vi "Mass_2_1_old.vi"() -> ()   [LabVIEW 2020]
uses:
  Support/Controls/Cmd_Mouse Popup.ctl
  Support/Controls/Clst_Initialize Input.ctl
  Support/Controls/Clst_Result inspec.ctl
  Support/Controls/Cmd_Var Data IO.ctl
  Variables/Global_Cal Info.vi
  <vilib>/express/express arith-compare/Formula/XNode/ExpressFormulaBlockNode.xnode
panel:
  in  "일괄\n변경":bool=TRUE
  in  "분동등급":string(combo)
  out "적용?":bool
  in  "다음 버튼":bool
  in  "이전 버튼":bool
  in  "제거":bool
  in  "적용":bool
  out "추가명목값":string caption="명목값"
  in  "추가":bool
  in  "추가문자열":string
  in  "시험분동 추가":i32(listbox)=24
  out "분해능":string caption="저울분해능 (g)"
  out "Data Out":string[][](table)
  out "단위":string
  out "명목질량":string
  in  "기기번호":string
  out "명목값":string
  in  "편심오차":string[][](table) caption="4. 저울 편심오차 시험"
  in  "측정횟수":i32(ring)=5 items=["5회"=5, "10회"=10]
  in  "시험분동밀도":string="8000" caption="분동밀도 (kg/㎤)"
  out "감도분동":string
  out "X=S-T":string[][](table)
  out "공기밀도":string
  out "Header2":string[][](table)
  in  "Measured":string[][](table) caption="3. 저울 지시값"
  out "Weight info":string[][](table) caption="2. 분동식별표기"
  out "Spec":string[][](table)
  in  "시험분동":i32(listbox)=-1
  in  "Spec 변경":bool
  out "제목":string
  out "에러 출력":errorcluster
  out "Condition":string[][](table)
  out "Atm Env":string[][](table) caption="1. 측정환경"
  out "Load?":bool
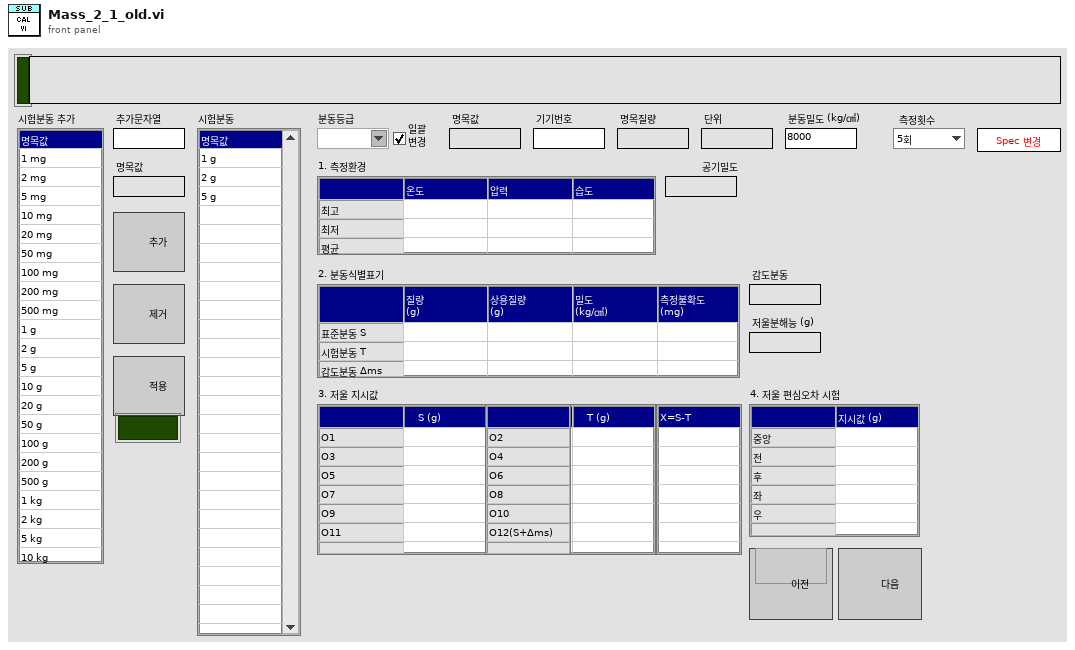
[diagram p1: front panel]
types:
  T1 = typedef "Cmd_Mouse Popup.ctl" = enum16{"활성화", "메뉴선택"}
  T2 = cluster{"Shift":bool, "Ctrl":bool, "Alt":bool, "Cmd":bool, "Opt":bool}
  T3 = typedef "Clst_Initialize Input.ctl" = cluster{"Initialize 1":cluster{"Condition":refnum<vi>[], "Spec":refnum<vi>[], "Measured":refnum<vi>[], "Resolution":refnum<vi>[], "Func_ext":string, "제목":refnum<vi>, "Measured_ADJ":refnum<vi>[]}, "Initialize 2":cluster{"문자열":refnum<vi>[], "콤보박스":refnum<vi>[], "링":refnum<vi>[], "열거형":refnum<vi>[], "테이블":refnum<vi>[], "여러열":refnum<vi>[], "디지털(DBL)":refnum<vi>[], "3D string":refnum<vi>[], "ctrl":refnum<vi>[], "boolean":refnum<vi>[]}}
  T4 = typedef "Cmd_Var Data IO.ctl" = enum16{"Condition", "Condition Default", "Condition_Temp", "Resolution", "Resolution Default", "Resolution Old", "Spec", "Spec Default", "Spec Old", "Spec Temp", "Result", "Result2", "Result3", "Result_Temp", "Result_ADJ", "Result_ADJ2", "STD1", "STD2", "STD3", "STD4", "STD5", "STD Temp", "CMC", "CMC Default"}
  T5 = typedef "Clst_Result inspec.ctl" = cluster{"분해능":string, "문자열 1":string, "문자열 2":string, "숫자형 1":i32, "숫자형 2":i32, "숫자형 3":dbl, "문자배열 1D":string[], "문자배열 2D":string[][], "문자배열 3D":string[][][], "문자배열 4D":string[][][][], "불리언 1D":bool[]}
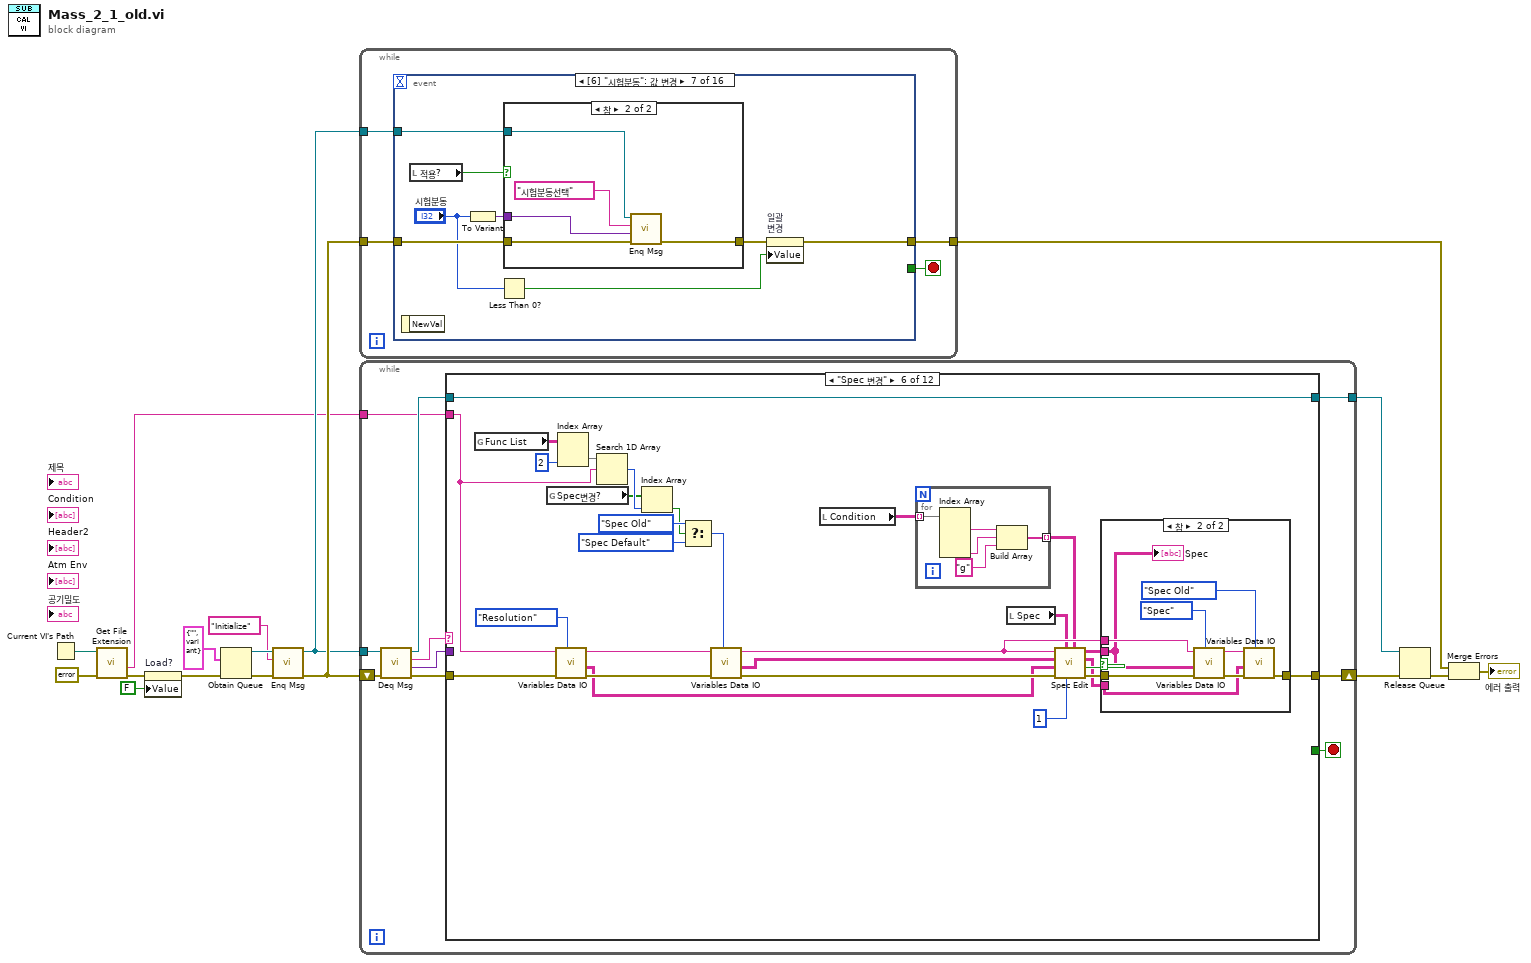
[diagram p0: block diagram]
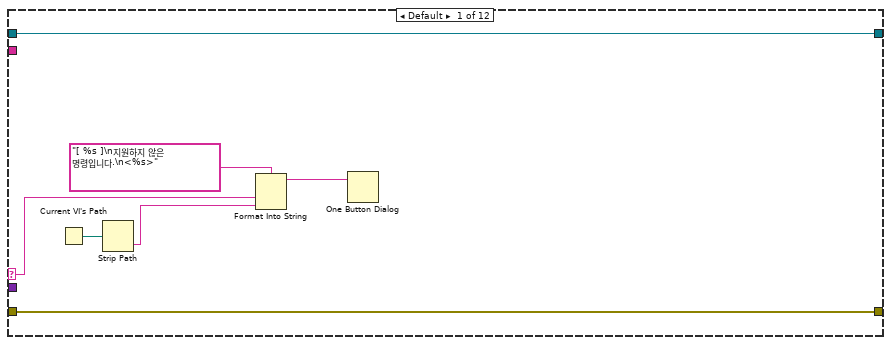
[diagram p2: hidden frame]
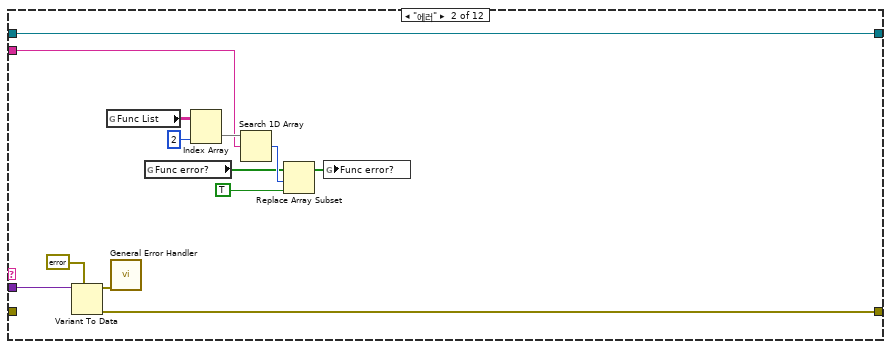
[diagram p3: hidden frame]
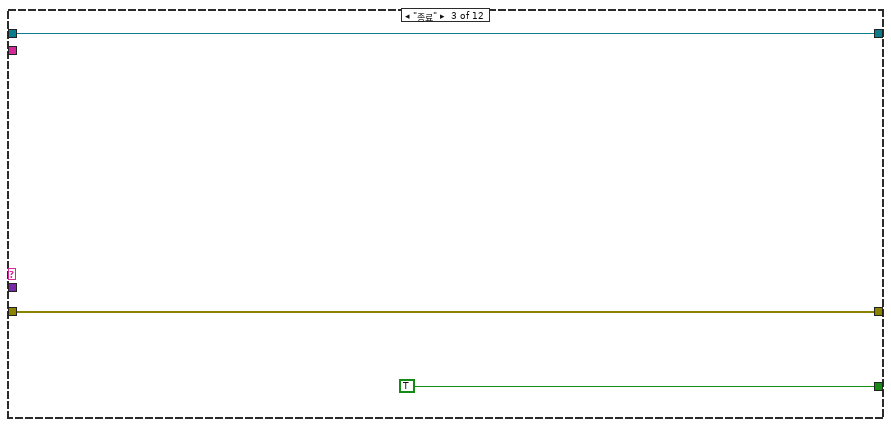
[diagram p4: hidden frame]
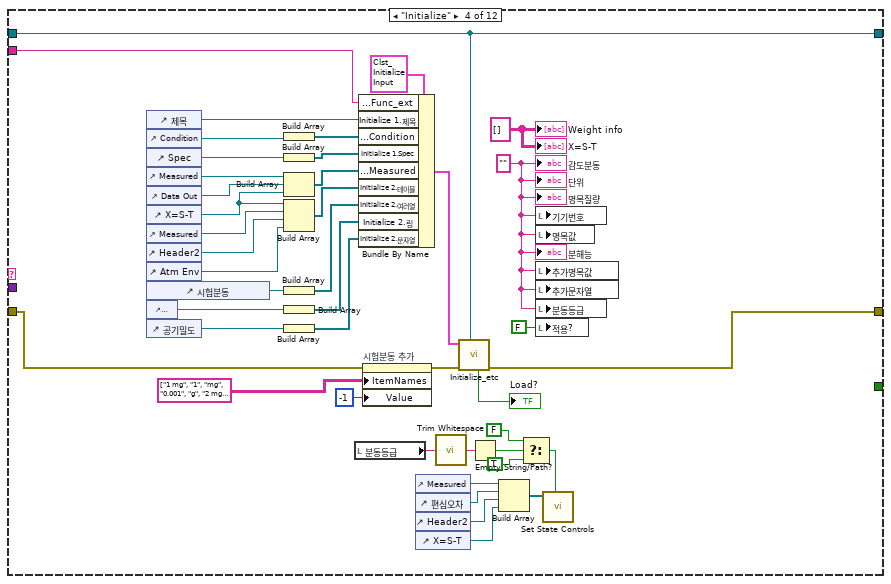
[diagram p5: hidden frame]
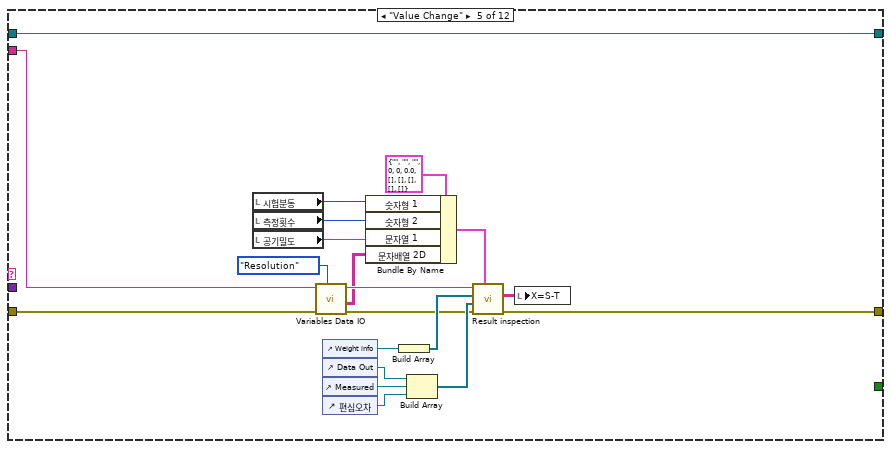
[diagram p6: hidden frame]
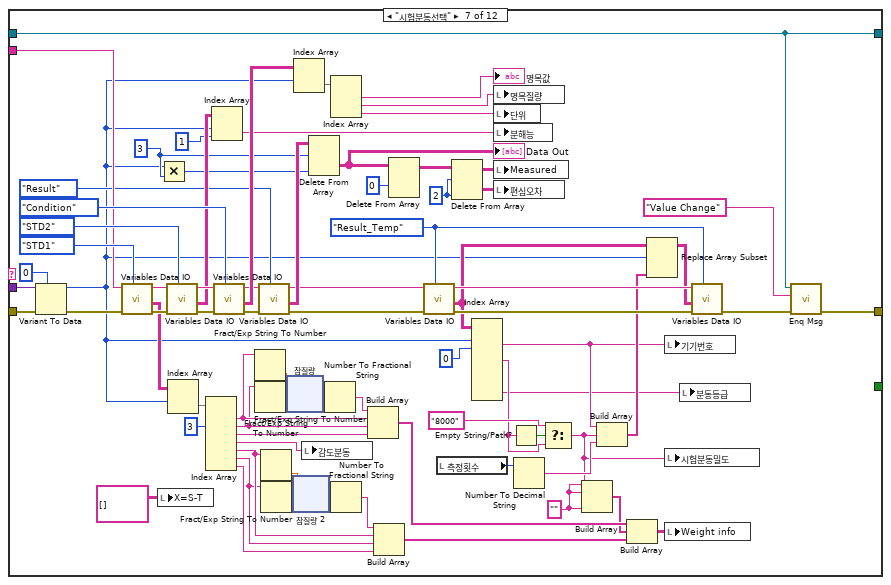
[diagram p8: hidden frame]
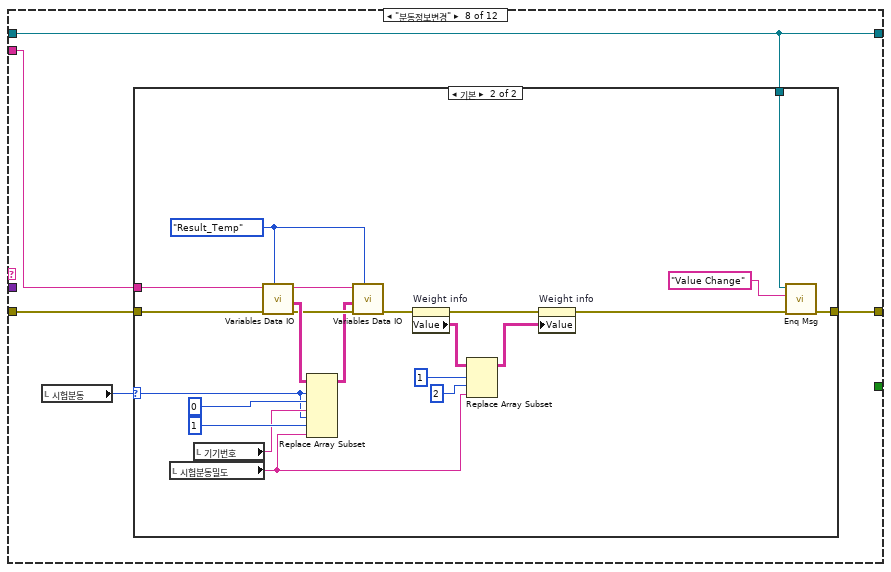
[diagram p9: hidden frame]
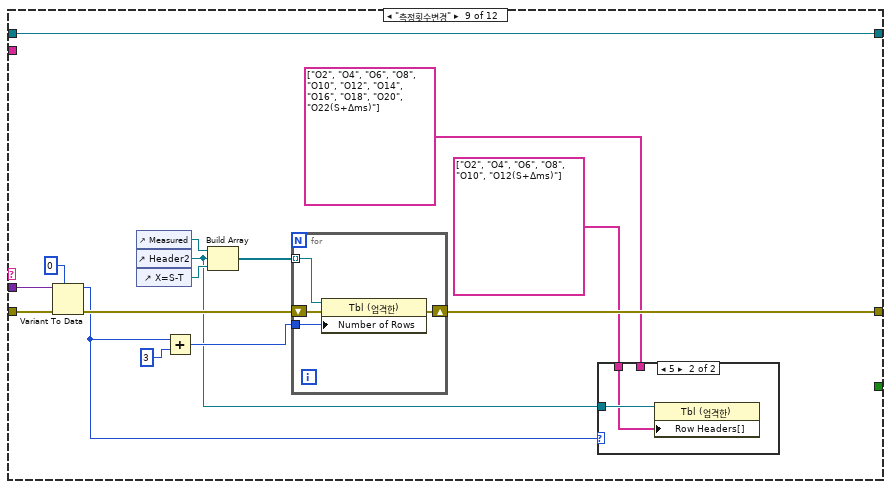
[diagram p11: hidden frame]
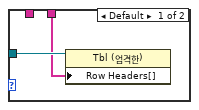
[diagram p12: hidden frame]
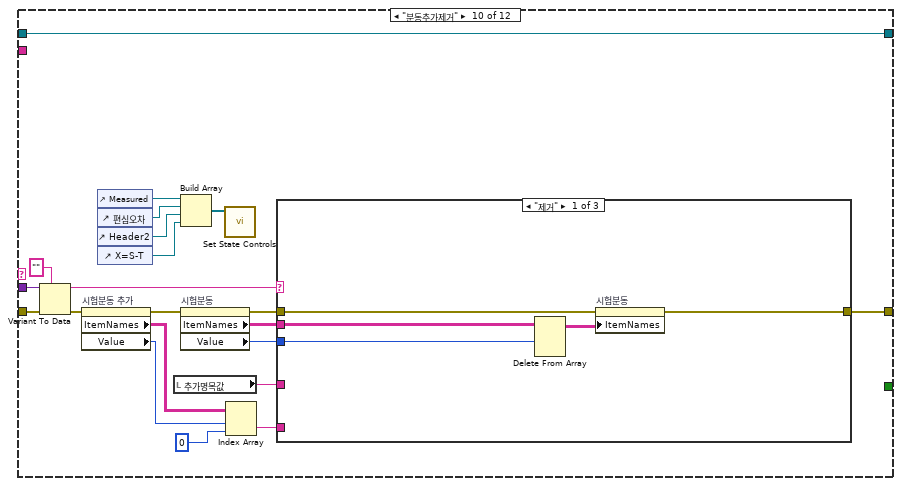
[diagram p13: hidden frame]
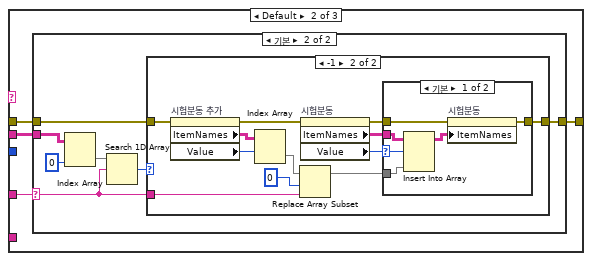
[diagram p14: hidden frame]
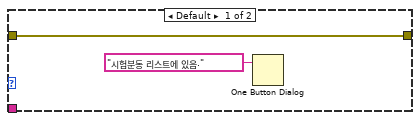
[diagram p16: hidden frame]
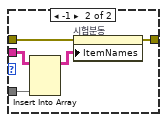
[diagram p17: hidden frame]
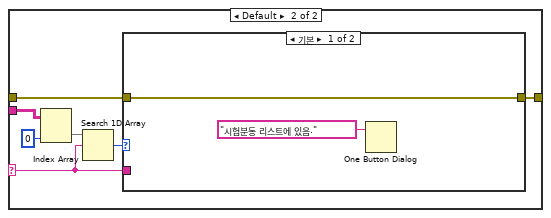
[diagram p19: hidden frame]
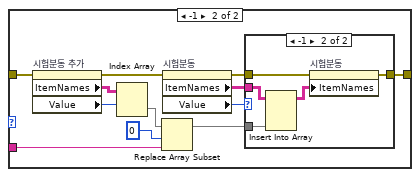
[diagram p20: hidden frame]
diagram:
  n1 = Current VI's Path() -> (path=w5:path)
  n2 = call <vilib>:"Get File Extension.vi"("error in (no error)"=errorcluster {"status"=FALSE, "code"=0, "source"=""} ("에러 상수"), "file"=w5) -> ("error out"=w3:errorcluster, "filename without extension"=w4:string)  [unwired: 5 in, 3 out]
  n3 = property on="Load?" class="Bool (엄격한)"(error in=w3, "Value"=FALSE ("Load?")) -> (error out=w2:errorcluster)  [unwired: 1 in, 1 out]
  n4 = Obtain Queue(element data type=cluster{"메세지":string, "값":variant} {"메세지"="", "값"=variant} ("Message Cluster"), error in (no error)=w2) -> (queue out=w14:refnum<queue>, error out=w16:errorcluster)  [unwired: 3 in, 1 out]
  n5 = call "Enq Msg.vi"("에러 입력(에러 없음)"=w16, "메세지"="Initialize", "큐 입력"=w14) -> ("에러 출력"=w15:errorcluster, "큐 출력"=w12:refnum<queue>)  [unwired: 7 in]
  n6 = while {
    tunnel: w15 -> [w19]
    tunnel: w12 -> [w20]
    tunnel: [w18] -> w9
    stop <- w21 stop-if-true
    n7 = event shown="[6] \"시험분동\": 값 변경" {
      selector: _ -> [_ _ _ _ _ _ _ _ _ _ _ _ _ _ _ _]
      dyn-events: _ -> [_ _ _ _ _ _ _ _ _ _ _ _ _ _ _ _]
      timeout: _ -> [_ _ _ _ _ _ _ _ _ _ _ _ _ _ _ _]
      tunnel: [w26 _ _ _ _ _ _ _ _ _ _ _ _ _ _ _] -> w21
      tunnel: w20 -> [w24 w29 _ w36 _ w49 w58 _ w79 w102 w119 _ w136 w141 w155 w157]
      tunnel: w19 -> [w25 w30 w33 w41 w48 w51 w60 w72 w81 w96 w121 w130 w138 w148 w153 w156]
      tunnel: [w22 w28 w32 w35 w47 w50 w54 w72 w80 w104 w120 w125 w137 w140 w154 w158] -> w18
      event Panel Close? {
        w26 = TRUE ("버림?")
        n8 = event-data() -> ()  [unwired: 1 in, 1 out]
        n9 = call "Enq Msg.vi"("에러 입력(에러 없음)"=w25, "메세지"="종료", "큐 입력"=w24) -> ("에러 출력"=w22:errorcluster)  [unwired: 7 in, 1 out]
        n10 = event-data("Discard?"=w26) -> ()  [unwired: 1 in, 1 out]
      }
      event "Measured", "편심오차": Value Change {
        n11 = event-data() -> ()  [unwired: 1 in, 3 out]
        n12 = call "Enq Msg.vi"("에러 입력(에러 없음)"=w30, "메세지"="Value Change", "큐 입력"=w29) -> ("에러 출력"=w28:errorcluster)  [unwired: 7 in, 1 out]
      }
      event "Measured", "편심오차": Shortcut Menu Activation? {
        n13 = event-data() -> ("MenuRef"=w31:refnum<k9>)  [unwired: 1 in]
        n14 = call "Mouse PopUp Control.vi"("type"=Cmd_Mouse_Popup."활성화", "error in"=w33, "메뉴 참조"=w31) -> ("error out"=w32:errorcluster)  [unwired: 8 in]
        n15 = event-data() -> ()  [unwired: 2 in, 1 out]
      }
      event "Measured", "편심오차": Shortcut Menu Selection (User) {
        n16 = event-data() -> ("CtlRef"=w39:refnum<vi>, "ItemTag"=w40:string)  [unwired: 1 in]
        n17 = call "Mouse PopUp Control.vi"("type"=Cmd_Mouse_Popup."메뉴선택", "error in"=w41, "아이템 태그"=w40, "Tbl 참조 번호"=w39) -> ("error out"=w37:errorcluster)  [unwired: 7 in]
        n18 = call "Enq Msg.vi"("에러 입력(에러 없음)"=w37, "메세지"="Value Change", "큐 입력"=w36) -> ("에러 출력"=w35:errorcluster)  [unwired: 7 in, 1 out]
      }
      event "Measured", "편심오차", "Condition": Key Down; "Measured", "편심오차", "Condition": Key Repeat {
        n19 = event-data() -> ("PlatMods"=w43:T2, "ScanCode"=w46:i16, "Mods.Num Pad"=w45:bool, "CtlRef"=w44:refnum<vi>)  [unwired: 1 in]
        n20 = call "Cursor Control.vi"("플랫폼 조합키"=w43, "참조"=w44, "Num Pad"=w45, "ScanCode"=w46, "error in"=w48) -> ("error out"=w47:errorcluster)  [unwired: 5 in, 1 out]
      }
      event "Spec 변경": Value Change {
        n21 = event-data() -> ()  [unwired: 1 in, 1 out]
        n22 = call "Enq Msg.vi"("에러 입력(에러 없음)"=w51, "메세지"="Spec 변경", "큐 입력"=w49) -> ("에러 출력"=w50:errorcluster)  [unwired: 7 in, 1 out]
      }
      event "시험분동": Value Change {
        n23 = event-data() -> ()  [unwired: 1 in, 1 out]
        n24 = local read "적용?"() -> (w57:bool)
        n25 = To Variant(anything="시험분동") -> (Variant=w59:variant)
        n26 = Less Than 0?(x="시험분동") -> (x < 0?=w53:bool)
        n27 = case shown="참" w57 {
          tunnel: w60 -> [w66 w70]
          tunnel: [w66 w69] -> w55
          tunnel: w59 -> [_ w68]
          tunnel: w58 -> [_ w67]
          frame False {
            n28 = control-ref of="Measured"() -> (w62:refnum<vi>)
            n29 = control-ref of="편심오차"() -> (w61:refnum<vi>)
            n30 = control-ref of="Header2"() -> (w64:refnum<vi>)
            n31 = control-ref of="X=S-T"() -> (w65:refnum<vi>)
            n32 = Build Array(w62, w61, w64, w65) -> (w63:refnum<vi>[])
            n33 = call "Set State Controls.vi"("컨트롤 참조 배열 in"=w63) -> ()  [unwired: 9 in, 2 out]
          }
          frame True {
            n34 = call "Enq Msg.vi"("에러 입력(에러 없음)"=w70, "값"=w68, "메세지"="시험분동선택", "큐 입력"=w67) -> ("에러 출력"=w69:errorcluster)  [unwired: 6 in, 1 out]
          }
        }
        n35 = property on="일괄\n변경" class="Bool (엄격한)"(error in=w55, "Value"=w53) -> (error out=w54:errorcluster)  [unwired: 1 in, 1 out]
      }
      event "시험분동": Drag Ended {
        n36 = event-data() -> ()  [unwired: 1 in, 4 out]
        n37 = control-ref of="Measured"() -> (w74:refnum<vi>)
        n38 = control-ref of="편심오차"() -> (w73:refnum<vi>)
        n39 = control-ref of="Header2"() -> (w76:refnum<vi>)
        n40 = control-ref of="X=S-T"() -> (w77:refnum<vi>)
        n41 = local write "적용?"(FALSE ("적용?")) -> ()
        n42 = Build Array(w74, w73, w76, w77) -> (w75:refnum<vi>[])
        n43 = call "Set State Controls.vi"("컨트롤 참조 배열 in"=w75) -> ()  [unwired: 9 in, 2 out]
      }
      event "시험분동": Double Click {
        n44 = event-data() -> ()  [unwired: 1 in, 1 out]
        n45 = local read "적용?"() -> (w82:bool)
        n46 = case shown="거짓" w82 {
          tunnel: w81 -> [w84 w89]
          tunnel: [w86 w89] -> w80
          tunnel: w79 -> [w85 _]
          frame False {
            n47 = To Variant(anything="제거") -> (Variant=w87:variant)
            n48 = call "Enq Msg.vi"("에러 입력(에러 없음)"=w84, "값"=w87, "메세지"="분동추가제거", "큐 입력"=w85) -> ("에러 출력"=w86:errorcluster)  [unwired: 6 in, 1 out]
          }
          frame True {
          }
        }
      }
      event "이전 버튼", "다음 버튼": Value Change {
        n49 = event-data() -> ()  [unwired: 1 in, 1 out]
        n50 = property on="시험분동" class="MCListbox (엄격한)"(error in=w96) -> (error out=w95:errorcluster, "Value"=w94:i32, "ItemNames"=w93:string[][])  [unwired: 1 in, 1 out]
        n51 = Build Array("이전 버튼", "다음 버튼") -> (w99:bool[])
        n52 = Array Size(array=w93) -> (size(s)=w92:i32[])
        n53 = Boolean Array To Number(Boolean array=w99) -> (number=w98:u32)
        n54 = Index Array(array=w92) -> (element=w91:i32)  [unwired: 1 in]
        n55 = Decrement(x=w91) -> (x-1=w90:i32)
        n56 = case shown="2" w98 {
          tunnel: w94 -> [w106 w110 w116]
          tunnel: [w106 w107 w115] -> w97
          tunnel: w90 -> [_ _ w113]
          frame Default {
          }
          frame 1 {
            n57 = Less Or Equal To 0?(x=w110) -> (x <= 0?=w111:bool)
            n58 = Decrement(x=w110) -> (x-1=w109:i32)
            n59 = Select(t=0, s=w111, f=w109) -> (s? t:f=w107:i32)
          }
          frame 2 {
            n60 = Increment(x=w116) -> (x+1=w114:i32)
            n61 = Less Or Equal?(x=w114, y=w113) -> (x <= y?=w112:bool)
            n62 = Select(t=w114, s=w112, f=w116) -> (s? t:f=w115:i32)
          }
        }
        n63 = local write "시험분동"(w97) -> ()
        n64 = To Variant(anything=w97) -> (Variant=w103:variant)
        n65 = call "Enq Msg.vi"("에러 입력(에러 없음)"=w95, "값"=w103, "메세지"="시험분동선택", "큐 입력"=w102) -> ("에러 출력"=w104:errorcluster)  [unwired: 6 in, 1 out]
      }
      event "측정횟수": Value Change {
        n66 = event-data() -> ()  [unwired: 1 in, 1 out]
        n67 = To Variant(anything="측정횟수") -> (Variant=w118:variant)
        n68 = call "Enq Msg.vi"("에러 입력(에러 없음)"=w121, "값"=w118, "메세지"="측정횟수변경", "큐 입력"=w119) -> ("에러 출력"=w120:errorcluster)  [unwired: 6 in, 1 out]
      }
      event "시험분동 추가", "추가문자열": Value Change {
        n69 = event-data() -> ()  [unwired: 1 in, 1 out]
        n70 = property on="시험분동 추가" class="MCListbox (엄격한)"(error in=w130) -> (error out=w125:errorcluster, "ItemNames"=w129:string[][])  [unwired: 1 in, 1 out]
        n71 = Index Array(array=w129, index (row) #1="시험분동 추가", index (row) #2="시험분동 추가", index (col) #2=0 ("비활성화된 인덱스 (열)")) -> (element #2=w126:string)  [unwired: 1 in, 1 out]
        n72 = case shown="기본" "추가문자열" {
          selector: "추가문자열" -> [_ w132]
          tunnel: w126 -> [w131 w134]
          tunnel: [w131 w133] -> w124
          frame "" {
          }
          frame Default {
            n73 = Format Into String(format string="%s (%s)" ("포맷 문자열"), w134, w132) -> (resulting string=w133:string)  [unwired: 2 in, 1 out]
          }
        }
        "추가명목값" <- w124
      }
      event "기기번호", "시험분동밀도": Value Change {
        n74 = event-data() -> ()  [unwired: 1 in, 3 out]
        n75 = call "Enq Msg.vi"("에러 입력(에러 없음)"=w138, "메세지"="분동정보변경", "큐 입력"=w136) -> ("에러 출력"=w137:errorcluster)  [unwired: 7 in, 1 out]
      }
      event "추가", "제거": Value Change; "시험분동 추가": Double Click {
        n76 = event-data() -> ("CtlRef"=w147:refnum<vi>)  [unwired: 1 in]
        n77 = property class="Ctl"(reference=w147, error in=w148) -> (error out=w143:errorcluster, "Label.Text"=w142:string)  [unwired: 1 out]
        n78 = To Variant(anything=w142) -> (Variant=w144:variant)
        n79 = call "Enq Msg.vi"("에러 입력(에러 없음)"=w143, "값"=w144, "메세지"="분동추가제거", "큐 입력"=w141) -> ("에러 출력"=w140:errorcluster)  [unwired: 6 in, 1 out]
        "적용?" <- FALSE ("적용?")
      }
      event "적용": Value Change {
        n80 = event-data() -> ()  [unwired: 1 in, 1 out]
        n81 = property on="시험분동" class="MCListbox (엄격한)"(error in=w153, "Value"=-1 ("시험분동")) -> (error out=w151:errorcluster)  [unwired: 1 in, 1 out]
        n82 = local write "적용?"(TRUE ("적용?")) -> ()
        n83 = call "Enq Msg.vi"("에러 입력(에러 없음)"=w151, "메세지"="분동추가적용", "큐 입력"=w155) -> ("에러 출력"=w154:errorcluster)  [unwired: 7 in, 1 out]
      }
      event "분동등급": Value Change {
        n84 = event-data() -> ()  [unwired: 1 in, 1 out]
        n85 = call "Enq Msg.vi"("에러 입력(에러 없음)"=w156, "메세지"="분동등급변경", "큐 입력"=w157) -> ("에러 출력"=w158:errorcluster)  [unwired: 7 in, 1 out]
      }
    }
  }
  n86 = while {
    shift-right: [w169] -> w11
    shift-left: w15 -> [w168]
    tunnel: w12 -> [w166]
    tunnel: [w161] -> w10
    tunnel: w4 -> [w160]
    stop <- w162 stop-if-true
    n87 = call "Deq Msg.vi"("에러 입력(에러 없음)"=w168, "큐 입력"=w166) -> ("에러 출력"=w167:errorcluster, "값"=w163:variant, "메세지"=w165:string, "큐 출력"=w164:refnum<queue>)  [unwired: 6 in]
    n88 = case shown="\"Spec 변경\"" w165 {
      selector: w165 -> [w172 _ _ _ _ _ _ _ _ _ _ _]
      tunnel: w167 -> [w176 _ w192 w216 w240 w277 w376 w401 w432 w457 w582 w627]
      tunnel: [w176 w186 w192 w222 w251 w281 w301 w400 w435 w458 w578 w631] -> w169
      tunnel: w164 -> [w175 w185 w190 w221 w255 w283 w300 w397 w439 w468 w597 w646]
      tunnel: w163 -> [_ w187 _ _ _ _ w375 _ w433 w456 _ _]
      tunnel: [_ _ TRUE ("버림?") _ _ _ _ _ _ _ _ _] -> w162
      tunnel: [w175 w185 w190 w221 w255 w283 w300 w397 w439 w468 w597 w646] -> w161
      tunnel: w160 -> [_ w177 _ w225 w238 w259 w353 w399 _ _ w581 w635]
      frame Default {
        n89 = Current VI's Path() -> (path=w171:path)
        n90 = Strip Path(path=w171) -> (name=w170:string)  [unwired: 1 out]
        n91 = Format Into String(format string="[ %s ]\n지원하지 않은 명령입니다.\n<%s>" ("메시지"), w172, w170) -> (resulting string=w173:string)  [unwired: 2 in, 1 out]
        n92 = One Button Dialog(message=w173) -> ()  [unwired: 1 in, 1 out]
      }
      frame "에러" {
        n93 = Variant To Data(type=errorcluster {"status"=FALSE, "code"=0, "source"=""} ("에러 출력"), Variant=w187) -> (data=w189:errorcluster, error out=w186:errorcluster)  [unwired: 1 in]
        n94 = global read "Global_Cal Info.vi" "Func List"() -> (w179:string[][])
        n95 = call <vilib>:"General Error Handler.vi"("error in (no error)"=w189) -> ()  [unwired: 10 in, 5 out]
        n96 = global read "Global_Cal Info.vi" "Func error?"() -> (w182:bool[])
        n97 = Index Array(array=w179, index (col)=2 ("비활성화된 인덱스 (열)")) -> (element=w180:string[])  [unwired: 1 in]
        n98 = Search 1D Array(1D array=w180, element=w177) -> (index of element=w183:i32)  [unwired: 1 in]
        n99 = Replace Array Subset(array=w182, new element=TRUE ("새 원소/부분배열"), index=w183) -> (w184:bool[])
        n100 = global write "Global_Cal Info.vi" "Func error?"(w184) -> ()
      }
      frame "종료" {
      }
      frame "Initialize" {
        w220 = string[][] [] ("Weight info")
        w194 = "" ("감도 분동")
        n101 = control-ref of="제목"() -> (w228:refnum<vi>)
        n102 = control-ref of="Condition"() -> (w233:refnum<vi>)
        n103 = control-ref of="Spec"() -> (w227:refnum<vi>)
        n104 = control-ref of="Measured"() -> (w230:refnum<vi>)
        n105 = control-ref of="Data Out"() -> (w196:refnum<vi>)
        n106 = control-ref of="X=S-T"() -> (w195:refnum<vi>)
        n107 = control-ref of="Measured"() -> (w218:refnum<vi>)
        n108 = control-ref of="Header2"() -> (w217:refnum<vi>)
        n109 = control-ref of="Atm Env"() -> (w209:refnum<vi>)
        n110 = control-ref of="시험분동"() -> (w224:refnum<vi>)
        n111 = control-ref of="측정횟수"() -> (w212:refnum<vi>)
        n112 = control-ref of="공기밀도"() -> (w211:refnum<vi>)
        n113 = Build Array(w233) -> (w232:refnum<vi>[])
        n114 = Build Array(w227) -> (w226:refnum<vi>[])
        n115 = Build Array(w230, w196, w195) -> (w231:refnum<vi>[])
        n116 = Build Array(w195, w218, w217, w209) -> (w229:refnum<vi>[])
        n117 = Build Array(w224) -> (w223:refnum<vi>[])
        n118 = Build Array(w212) -> (w219:refnum<vi>[])
        n119 = Build Array(w211) -> (w210:refnum<vi>[])
        n120 = local read "분동등급"() -> (w203:string)
        n121 = Bundle By Name(cluster=T3 {"Initialize 1"={"Condition"=[], "Spec"=[], "Measured"=[], "Resolution"=[], "Func_ext"="", "제목"=refnum, "Measured_ADJ"=[]}, "Initialize 2"={"문자열"=[], "콤보박스"=[], "링"=[], "열거형"=[], "테이블"=[], "여러열"=[], "디지털(DBL)"=[], "3D string"=[], "ctrl"=[], "boolean"=[]}} ("입력 클러스터"), "Initialize 1.Func_ext"=w225, "Initialize 1.제목"=w228, "Initialize 1.Condition"=w232, "Initialize 1.Spec"=w226, "Initialize 1.Measured"=w231, "Initialize 2.테이블"=w229, "Initialize 2.여러열"=w223, "Initialize 2.링"=w219, "Initialize 2.문자열"=w210) -> (w234:T3)
        n122 = property on="시험분동 추가" class="MCListbox (엄격한)"(error in=w216, "ItemNames"=string[][] [["1 mg", "1", "mg", "0.001", "g"], ["2 mg", "2", "mg", "0.002", "g"], ["5 mg", "5", "mg", "0.005", "g"], ["10 mg", "10", "mg", "0.01", "g"], ["20 mg", "20", "mg", "0.02", "g"], ["50 mg", "50", "mg", "0.05", "g"], ["100 mg", "100", "mg", "0.1", "g"], ["200 mg", "200", "mg", "0.2", "g"], ["500 mg", "500", "mg", "0.5", "g"], ["1 g", "1", "g", "1", "g"], ["2 g", "2", "g", "2", "g"], ["5 g", "5", "g", "5", "g"], ["10 g", "10", "g", "10", "g"], ["20 g", "20", "g", "20", "g"], ["50 g", "50", "g", "50", "g"], ["100 g", "100", "g", "100", "g"], ["200 g", "200", "g", "200", "g"], ["500 g", "500", "g", "500", "g"], ["1 kg", "1", "kg", "1000", "g"], ["2 kg", "2", "kg", "2000", "g"], ["5 kg", "5", "kg", "5000", "g"], ["10 kg", "10", "kg", "10000", "g"], ["20 kg", "20", "kg", "20000", "g"]] ("테이블 컨트롤"), "Value"=-1 ("시험분동 추가")) -> (error out=w215:errorcluster)  [unwired: 1 in, 1 out]
        n123 = control-ref of="Measured"() -> (w205:refnum<vi>)
        n124 = control-ref of="편심오차"() -> (w206:refnum<vi>)
        n125 = control-ref of="Header2"() -> (w207:refnum<vi>)
        n126 = control-ref of="X=S-T"() -> (w208:refnum<vi>)
        n127 = call <vilib>:"Trim Whitespace.vi"("string"=w203) -> ("trimmed string"=w202:string)  [unwired: 1 in]
        n128 = call "Initialize_etc.vi"("큐 입력"=w221, "error in"=w215, "입력 클러스터"=w234) -> ("error out"=w222:errorcluster, "Load?"=→"Load?":bool)  [unwired: 6 in, 1 out]
        n129 = Empty String/Path?(string/path=w202) -> (empty?=w201:bool)
        n130 = Build Array(w205, w206, w207, w208) -> (w204:refnum<vi>[])
        n131 = Select(t=FALSE, s=w201, f=TRUE) -> (s? t:f=w198:bool)
        n132 = local write "기기번호"(w194) -> ()
        n133 = local write "명목값"(w194) -> ()
        n134 = local write "추가명목값"(w194) -> ()
        n135 = local write "추가문자열"(w194) -> ()
        n136 = local write "분동등급"(w194) -> ()
        n137 = local write "적용?"(FALSE ("적용?")) -> ()
        n138 = call "Set State Controls.vi"("활성화 (F)"=w198, "컨트롤 참조 배열 in"=w204) -> ()  [unwired: 8 in, 2 out]
        "감도분동" <- w194
        "Weight info" <- w220
        "단위" <- w194
        "명목질량" <- w194
        "X=S-T" <- w220
        "분해능" <- w194
      }
      frame "Value Change" {
        n139 = local read "시험분동"() -> (w248:i32)
        n140 = local read "측정횟수"() -> (w247:i32)
        n141 = local read "공기밀도"() -> (w246:string)
        n142 = call "Variables Data IO.vi"("Select"=Cmd_Var_Data_IO."Resolution", "error in"=w240, "Func_ext"=w238) -> ("error out"=w239:errorcluster, "Data Out"=w236:string[][], "Func_ext Out"=w237:string)  [unwired: 6 in]
        n143 = control-ref of="Weight info"() -> (w250:refnum<vi>)
        n144 = control-ref of="Data Out"() -> (w243:refnum<vi>)
        n145 = control-ref of="Measured"() -> (w242:refnum<vi>)
        n146 = control-ref of="편심오차"() -> (w244:refnum<vi>)
        n147 = Bundle By Name(cluster=T5 {"분해능"="", "문자열 1"="", "문자열 2"="", "숫자형 1"=0, "숫자형 2"=0, "숫자형 3"=0.0, "문자배열 1D"=[], "문자배열 2D"=[], "문자배열 3D"=[], "문자배열 4D"=[], "불리언 1D"=[]} ("입력 클러스터"), "숫자형 1"=w248, "숫자형 2"=w247, "문자열 1"=w246, "문자배열 2D"=w236) -> (w252:T5)
        n148 = Build Array(w250) -> (w254:refnum<vi>[])
        n149 = Build Array(w243, w242, w244) -> (w249:refnum<vi>[])
        n150 = call "Result inspection.vi"("입력 클러스터"=w252, "error in"=w239, "Ref. Data (excluded)"=w249, "Ref. Data (Inspection)"=w254, "Func ext"=w237) -> ("error out"=w251:errorcluster, "Data (spec 미적용)"=w245:string[][])  [unwired: 3 in, 2 out]
        n151 = local write "X=S-T"(w245) -> ()
      }
      frame "Spec 변경" {
        n152 = global read "Global_Cal Info.vi" "Func List"() -> (w264:string[][])
        n153 = global read "Global_Cal Info.vi" "Spec변경?"() -> (w260:bool[])
        n154 = call "Variables Data IO.vi"("Select"=Cmd_Var_Data_IO."Resolution", "error in"=w277, "Func_ext"=w259) -> ("error out"=w276:errorcluster, "Data Out"=w270:string[][], "Func_ext Out"=w275:string)  [unwired: 6 in]
        n155 = Index Array(array=w264, index (col)=2 ("비활성화된 인덱스 (열)")) -> (element=w262:string[])  [unwired: 1 in]
        n156 = Search 1D Array(1D array=w262, element=w259) -> (index of element=w261:i32)  [unwired: 1 in]
        n157 = Index Array(array=w260, index=w261) -> (element=w265:bool)
        n158 = Select(t=Cmd_Var_Data_IO."Spec Old" ("Select"), s=w265, f=Cmd_Var_Data_IO."Spec Default" ("Select")) -> (s? t:f=w258:T4)
        n159 = call "Variables Data IO.vi"("Select"=w258, "error in"=w276, "Func_ext"=w275) -> ("error out"=w278:errorcluster, "Data Out"=w269:string[][], "Func_ext Out"=w271:string)  [unwired: 6 in]
        n160 = local read "Condition"() -> (w257:string[][])
        n161 = for {
          tunnel: w257 -> [w288] mode=indexing
          tunnel: [w287] -> w256 mode=indexing
          n162 = Index Array(array=w288) -> (element #1=w286:string, element #4=w285:string)  [unwired: 4 in, 2 out]
          n163 = Build Array(w286, w285, "g" ("원소")) -> (w287:string[])
        }
        n164 = local read "Spec"() -> (w268:string[][])
        n165 = call "Spec Edit.vi"("Condition"=w256, "열번호(기준값)"=1 ("기준열(0)"), "Spec Value"=w268, "에러 입력(에러 없음)"=w278, "Resolution"=w270, "Spec Default"=w269, "Func_ext"=w271) -> ("에러 출력"=w282:errorcluster, "변경?"=w279:bool, "Spec Default out"=w273:string[][], "Spec 출력"=w280:string[][])  [unwired: 1 in]
        n166 = case shown="참" w279 {
          tunnel: w282 -> [w289 w297]
          tunnel: [w289 w293] -> w281
          tunnel: w280 -> [_ w295]
          tunnel: w271 -> [_ w296]
          tunnel: w273 -> [_ w291]
          frame False {
          }
          frame True {
            n167 = call "Variables Data IO.vi"("Select"=Cmd_Var_Data_IO."Spec", "error in"=w297, "Data In"=w295, "Func_ext"=w296) -> ("error out"=w294:errorcluster, "Func_ext Out"=w292:string)  [unwired: 5 in, 1 out]
            n168 = call "Variables Data IO.vi"("Select"=Cmd_Var_Data_IO."Spec Old", "error in"=w294, "Data In"=w291, "Func_ext"=w292) -> ("error out"=w293:errorcluster)  [unwired: 5 in, 2 out]
            "Spec" <- w295
          }
        }
      }
      frame "시험분동선택" {
        w312 = 2 ("비활성화된 인덱스 (열)")
        w321 = Cmd_Var_Data_IO."Result_Temp" ("Select")
        w330 = "" ("원소")
        w332 = 3 ("길이")
        n169 = Variant To Data(error in=w376, type=0, Variant=w375) -> (data=w310:i32, error out=w352:errorcluster)
        n170 = call "Variables Data IO.vi"("Select"=Cmd_Var_Data_IO."STD1", "error in"=w352, "Func_ext"=w353) -> ("error out"=w360:errorcluster, "Data Out"=w350:string[][], "Func_ext Out"=w359:string)  [unwired: 6 in]
        n171 = local write "X=S-T"(string[][] [] ("X=S-T")) -> ()
        n172 = Multiply(x=w310, y=w332) -> (x*y=w331:i32)
        n173 = call "Variables Data IO.vi"("Select"=Cmd_Var_Data_IO."STD2", "error in"=w360, "Func_ext"=w359) -> ("error out"=w351:errorcluster, "Data Out"=w339:string[][], "Func_ext Out"=w340:string)  [unwired: 6 in]
        n174 = Index Array(array=w350, index (row)=w310) -> (element=w349:string[])  [unwired: 1 in]
        n175 = Index Array(array=w349, index #1=3 ("인덱스")) -> (element #1=w347:string, element #2=w346:string, element #3=w345:string, element #4=w344:string, element #5=w343:string, element #6=w342:string, element #7=w341:string)  [unwired: 6 in]
        n176 = Index Array(array=w339, index (row)=w310, index (col)=1 ("비활성화된 인덱스 (열)")) -> (element=w337:string)
        n177 = call "Variables Data IO.vi"("Select"=Cmd_Var_Data_IO."Condition", "error in"=w351, "Func_ext"=w340) -> ("error out"=w336:errorcluster, "Data Out"=w357:string[][], "Func_ext Out"=w335:string)  [unwired: 6 in]
        n178 = Fract/Exp String To Number(string=w347) -> (number=w371:dbl)  [unwired: 3 in, 1 out]
        n179 = Fract/Exp String To Number(string=w346) -> (number=w370:dbl)  [unwired: 3 in, 1 out]
        n180 = call "Variables Data IO.vi"("Select"=Cmd_Var_Data_IO."Result", "error in"=w336, "Func_ext"=w335) -> ("error out"=w325:errorcluster, "Data Out"=w333:string[][], "Func_ext Out"=w323:string)  [unwired: 6 in]
        n181 = Fract/Exp String To Number(string=w343) -> (number=w366:dbl)  [unwired: 3 in, 1 out]
        n182 = Fract/Exp String To Number(string=w342) -> (number=w365:dbl)  [unwired: 3 in, 1 out]
        n183 = xnode ("참질량")("mc"=w371, "d"=w370) -> ("결과"=w369:dbl)  [unwired: 1 in, 1 out]
        n184 = xnode ("참질량 2")("mc"=w366, "d"=w365) -> ("결과"=w364:dbl)  [unwired: 1 in, 1 out]
        n185 = Index Array(array=w357, index (row)=w310) -> (element=w356:string[])  [unwired: 1 in]
        n186 = local write "감도분동"(w344) -> ()
        n187 = Delete From Array(array=w333, length=w332, index (col)=w331) -> (deleted portion=w317:string[][])  [unwired: 1 in, 1 out]
        "Data Out" <- w317
        n188 = Number To Fractional String(number=w369) -> (F-format string=w368:string)  [unwired: 3 in]
        n189 = Index Array(array=w356) -> (element #1=→"명목값":string, element #2=w355:string, element #3=w354:string)  [unwired: 3 in]
        n190 = Number To Fractional String(number=w364) -> (F-format string=w363:string)  [unwired: 3 in]
        n191 = Build Array(w368, w347, w346, w345) -> (w367:string[])
        n192 = Build Array(w363, w343, w342, w341) -> (w362:string[])
        n193 = Delete From Array(array=w317, index (row)=0 ("인덱스 (행)")) -> (array with subset deleted=w315:string[][])  [unwired: 2 in, 1 out]
        n194 = call "Variables Data IO.vi"("Select"=w321, "error in"=w325, "Func_ext"=w323) -> ("error out"=w324:errorcluster, "Data Out"=w311:string[][], "Func_ext Out"=w322:string)  [unwired: 6 in]
        n195 = local read "측정횟수"() -> (w327:i32)
        n196 = Delete From Array(array=w315, length=w312, index (col)=w312) -> (deleted portion=w313:string[][], array with subset deleted=w314:string[][])  [unwired: 1 in]
        n197 = Index Array(array=w311, index (row) #1=w310, index (col) #1=0 ("비활성화된 인덱스 (열)")) -> (element #1=w304:string, element #2=w305:string, element #4=w299:string)  [unwired: 6 in, 1 out]
        n198 = local write "명목질량"(w355) -> ()
        n199 = local write "단위"(w354) -> ()
        n200 = local write "분해능"(w337) -> ()
        n201 = local write "Measured"(w314) -> ()
        n202 = local write "편심오차"(w313) -> ()
        n203 = Empty String/Path?(string/path=w305) -> (empty?=w308:bool)
        n204 = Number To Decimal String(number=w327) -> (decimal integer string=w326:string)  [unwired: 1 in]
        n205 = Select(t="8000" ("원소"), s=w308, f=w305) -> (s? t:f=w306:string)
        n206 = Build Array(w330, w330, w306, w330) -> (w329:string[])
        n207 = Build Array(w304, w306, w326) -> (w320:string[])
        n208 = Build Array(w367, w329, w362) -> (w361:string[][])
        n209 = Replace Array Subset(array=w311, new element=w320, index (row)=w310) -> (w319:string[][])  [unwired: 1 in]
        n210 = local write "기기번호"(w304) -> ()
        n211 = local write "시험분동밀도"(w306) -> ()
        n212 = local write "Weight info"(w361) -> ()
        n213 = local write "분동등급"(w299) -> ()
        n214 = call "Variables Data IO.vi"("Select"=w321, "error in"=w324, "Data In"=w319, "Func_ext"=w322) -> ("error out"=w302:errorcluster)  [unwired: 5 in, 2 out]
        n215 = call "Enq Msg.vi"("에러 입력(에러 없음)"=w302, "메세지"="Value Change", "큐 입력"=w300) -> ("에러 출력"=w301:errorcluster)  [unwired: 7 in, 1 out]
      }
      frame "분동정보변경" {
        n216 = local read "시험분동"() -> (w398:i32)
        n217 = case shown="기본" w398 {
          selector: w398 -> [_ w403]
          tunnel: w401 -> [w402 w423]
          tunnel: [w402 w415] -> w400
          tunnel: w399 -> [_ w424]
          tunnel: w397 -> [_ w414]
          frame -1 {
          }
          frame Default {
            w417 = Cmd_Var_Data_IO."Result_Temp" ("Select")
            n218 = local read "시험분동밀도"() -> (w408:string)
            n219 = local read "기기번호"() -> (w404:string)
            n220 = call "Variables Data IO.vi"("Select"=w417, "error in"=w423, "Func_ext"=w424) -> ("error out"=w419:errorcluster, "Data Out"=w422:string[][], "Func_ext Out"=w418:string)  [unwired: 6 in]
            n221 = Replace Array Subset(array=w422, new element #1=w404, index (row) #1=w403, index (col) #1=0 ("비활성화된 인덱스 (열)"), new element #2=w408, index (row) #2=w403, index (col) #2=1 ("비활성화된 인덱스 (열)")) -> (w416:string[][])
            n222 = call "Variables Data IO.vi"("Select"=w417, "error in"=w419, "Data In"=w416, "Func_ext"=w418) -> ("error out"=w412:errorcluster)  [unwired: 5 in, 2 out]
            n223 = property on="Weight info" class="Tbl (엄격한)"(error in=w412) -> (error out=w407:errorcluster, "Value"=w411:string[][])  [unwired: 1 in, 1 out]
            n224 = Replace Array Subset(array=w411, new element=w408, index (row)=1 ("인덱스 (행)"), index (col)=2 ("비활성화된 인덱스 (열)")) -> (w406:string[][])
            n225 = property on="Weight info" class="Tbl (엄격한)"(error in=w407, "Value"=w406) -> (error out=w405:errorcluster)  [unwired: 1 in, 1 out]
            n226 = call "Enq Msg.vi"("에러 입력(에러 없음)"=w405, "메세지"="Value Change", "큐 입력"=w414) -> ("에러 출력"=w415:errorcluster)  [unwired: 7 in, 1 out]
          }
        }
      }
      frame "측정횟수변경" {
        n227 = Variant To Data(error in=w432, type=u32 0, Variant=w433) -> (data=w428:u32, error out=w431:errorcluster)
        n228 = control-ref of="Measured"() -> (w438:refnum<vi>)
        n229 = control-ref of="Header2"() -> (w427:refnum<vi>)
        n230 = control-ref of="X=S-T"() -> (w437:refnum<vi>)
        n231 = Add(x=w428, y=u32 3) -> (x+y=w430:u32)
        n232 = Build Array(w438, w427, w437) -> (w436:refnum<vi>[])
        n233 = for {
          tunnel: w436 -> [w445] mode=indexing
          shift-right: [w446] -> w435
          shift-left: w431 -> [w447]
          tunnel: w430 -> [w444]
          n234 = property class="Tbl (엄격한)"(reference=w445, error in=w447, "Number of Rows"=w444) -> (error out=w446:errorcluster)  [unwired: 1 out]
        }
        n235 = case shown="5" w428 {
          tunnel: w427 -> [w441 w443]
          tunnel: string[] ["O2", "O4", "O6", "O8", "O10", "O12", "O14", "O16", "O18", "O20", "O22(S+Δms)"] ("행 헤더 문자열[]") -> [w440 _]
          tunnel: string[] ["O2", "O4", "O6", "O8", "O10", "O12(S+Δms)"] ("행 헤더 문자열[]") -> [_ w442]
          frame Default {
            n236 = property class="Tbl (엄격한)"(reference=w441, "Row Headers[]"=w440) -> ()  [unwired: 1 in, 2 out]
          }
          frame 5 {
            n237 = property class="Tbl (엄격한)"(reference=w443, "Row Headers[]"=w442) -> ()  [unwired: 1 in, 2 out]
          }
        }
      }
      frame "분동추가제거" {
        n238 = Variant To Data(error in=w457, type="", Variant=w456) -> (data=w455:string, error out=w453:errorcluster)
        n239 = property on="시험분동 추가" class="MCListbox (엄격한)"(error in=w453) -> (error out=w452:errorcluster, "ItemNames"=w450:string[][], "Value"=w449:i32)  [unwired: 1 in, 1 out]
        n240 = control-ref of="Measured"() -> (w464:refnum<vi>)
        n241 = control-ref of="편심오차"() -> (w465:refnum<vi>)
        n242 = control-ref of="Header2"() -> (w466:refnum<vi>)
        n243 = control-ref of="X=S-T"() -> (w467:refnum<vi>)
        n244 = local read "추가명목값"() -> (w462:string)
        n245 = Build Array(w464, w465, w466, w467) -> (w463:refnum<vi>[])
        n246 = property on="시험분동" class="MCListbox (엄격한)"(error in=w452) -> (error out=w460:errorcluster, "ItemNames"=w459:string[][], "Value"=w461:i32)  [unwired: 1 in, 1 out]
        n247 = call "Set State Controls.vi"("컨트롤 참조 배열 in"=w463) -> ()  [unwired: 9 in, 2 out]
        n248 = Index Array(array=w450, index (row)=w449, index (col)=0 ("비활성화된 인덱스 (열)")) -> (element=w448:string)
        n249 = case shown="\"제거\"" w455 {
          tunnel: w459 -> [w472 w477 w514]
          tunnel: w460 -> [w470 w476 w513]
          tunnel: [w469 w475 w512] -> w458
          tunnel: w461 -> [w471 _ _]
          tunnel: w462 -> [_ w474 _]
          tunnel: w448 -> [_ _ w511]
          frame "제거" {
            n250 = Delete From Array(array=w472, index (row)=w471) -> (array with subset deleted=w473:string[][])  [unwired: 2 in, 1 out]
            n251 = property on="시험분동" class="MCListbox (엄격한)"(error in=w470, "ItemNames"=w473) -> (error out=w469:errorcluster)  [unwired: 1 in, 1 out]
          }
          frame Default {
            n252 = case shown="기본" w474 {
              selector: w474 -> [_ w479]
              tunnel: w477 -> [_ w485]
              tunnel: w476 -> [w478 w482]
              tunnel: [w478 w481] -> w475
              frame "" {
              }
              frame Default {
                n253 = Index Array(array=w485, index (col)=0 ("비활성화된 인덱스 (열)")) -> (element=w480:string[])  [unwired: 1 in]
                n254 = Search 1D Array(1D array=w480, element=w479) -> (index of element=w483:i32)  [unwired: 1 in]
                n255 = case shown="-1" w483 {
                  tunnel: w482 -> [w487 w497]
                  tunnel: [w487 w488] -> w481
                  tunnel: w479 -> [_ w491]
                  frame Default {
                    n256 = One Button Dialog(message="시험분동 리스트에 있음." ("메시지")) -> ()  [unwired: 1 in, 1 out]
                  }
                  frame -1 {
                    n257 = property on="시험분동 추가" class="MCListbox (엄격한)"(error in=w497) -> (error out=w494:errorcluster, "ItemNames"=w496:string[][], "Value"=w495:i32)  [unwired: 1 in, 1 out]
                    n258 = Index Array(array=w496, index (row)=w495) -> (element=w493:string[])  [unwired: 1 in]
                    n259 = Replace Array Subset(array=w493, new element=w491, index=0 ("인덱스")) -> (w490:string[])
                    n260 = property on="시험분동" class="MCListbox (엄격한)"(error in=w494) -> (error out=w498:errorcluster, "ItemNames"=w499:string[][], "Value"=w489:i32)  [unwired: 1 in, 1 out]
                    n261 = case shown="기본" w489 {
                      selector: w489 -> [w500 _]
                      tunnel: w499 -> [w505 w510]
                      tunnel: w498 -> [w504 w509]
                      tunnel: [w502 w507] -> w488
                      tunnel: w490 -> [w501 w506]
                      frame Default {
                        n262 = Insert Into Array(array=w505, index (row)=w500, new element=w501) -> (w503:string[][])  [unwired: 1 in]
                        n263 = property on="시험분동" class="MCListbox (엄격한)"(error in=w504, "ItemNames"=w503) -> (error out=w502:errorcluster)  [unwired: 1 in, 1 out]
                      }
                      frame -1 {
                        n264 = Insert Into Array(array=w510, new element=w506) -> (w508:string[][])  [unwired: 2 in]
                        n265 = property on="시험분동" class="MCListbox (엄격한)"(error in=w509, "ItemNames"=w508) -> (error out=w507:errorcluster)  [unwired: 1 in, 1 out]
                      }
                    }
                  }
                }
              }
            }
          }
          frame "시험분동 추가" {
            n266 = case shown="\"\"" w511 {
              selector: w511 -> [_ w516]
              tunnel: w514 -> [_ w522]
              tunnel: w513 -> [w515 w519]
              tunnel: [w515 w518] -> w512
              frame "" {
              }
              frame Default {
                n267 = Index Array(array=w522, index (col)=0 ("비활성화된 인덱스 (열)")) -> (element=w517:string[])  [unwired: 1 in]
                n268 = Search 1D Array(1D array=w517, element=w516) -> (index of element=w520:i32)  [unwired: 1 in]
                n269 = case shown="기본" w520 {
                  tunnel: w519 -> [w524 w534]
                  tunnel: [w524 w525] -> w518
                  tunnel: w516 -> [_ w528]
                  frame Default {
                    n270 = One Button Dialog(message="시험분동 리스트에 있음." ("메시지")) -> ()  [unwired: 1 in, 1 out]
                  }
                  frame -1 {
                    n271 = property on="시험분동 추가" class="MCListbox (엄격한)"(error in=w534) -> (error out=w531:errorcluster, "ItemNames"=w533:string[][], "Value"=w532:i32)  [unwired: 1 in, 1 out]
                    n272 = Index Array(array=w533, index (row)=w532) -> (element=w530:string[])  [unwired: 1 in]
                    n273 = Replace Array Subset(array=w530, new element=w528, index=0 ("인덱스")) -> (w527:string[])
                    n274 = property on="시험분동" class="MCListbox (엄격한)"(error in=w531) -> (error out=w535:errorcluster, "ItemNames"=w536:string[][], "Value"=w526:i32)  [unwired: 1 in, 1 out]
                    n275 = case shown="-1" w526 {
                      selector: w526 -> [w537 _]
                      tunnel: w536 -> [w542 w547]
                      tunnel: w535 -> [w541 w546]
                      tunnel: [w539 w544] -> w525
                      tunnel: w527 -> [w538 w543]
                      frame Default {
                        n276 = Insert Into Array(array=w542, index (row)=w537, new element=w538) -> (w540:string[][])  [unwired: 1 in]
                        n277 = property on="시험분동" class="MCListbox (엄격한)"(error in=w541, "ItemNames"=w540) -> (error out=w539:errorcluster)  [unwired: 1 in, 1 out]
                      }
                      frame -1 {
                        n278 = Insert Into Array(array=w547, new element=w543) -> (w545:string[][])  [unwired: 2 in]
                        n279 = property on="시험분동" class="MCListbox (엄격한)"(error in=w546, "ItemNames"=w545) -> (error out=w544:errorcluster)  [unwired: 1 in, 1 out]
                      }
                    }
                  }
                }
              }
            }
          }
        }
      }
      frame "분동추가적용" {
        w569 = Cmd_Var_Data_IO."Result_Temp" ("Select")
        w586 = Cmd_Var_Data_IO."Result" ("Select")
        n280 = property on="시험분동" class="MCListbox (엄격한)"(error in=w582) -> (error out=w561:errorcluster, "ItemNames"=w550:string[][])  [unwired: 1 in, 1 out]
        n281 = control-ref of="Spec"() -> (w595:refnum<vi>)
        n282 = control-ref of="Condition"() -> (w564:refnum<vi>)
        n283 = call "Table Initialize_2D.vi"("Table Ref"=w564, "Value"=w550, "에러 입력"=w561) -> ("에러 출력"=w560:errorcluster)  [unwired: 6 in, 2 out]
        n284 = control-ref of="Measured"() -> (w592:refnum<vi>)
        n285 = control-ref of="편심오차"() -> (w593:refnum<vi>)
        n286 = control-ref of="Header2"() -> (w590:refnum<vi>)
        n287 = control-ref of="X=S-T"() -> (w589:refnum<vi>)
        n288 = call "Variables Data IO.vi"("Select"=Cmd_Var_Data_IO."Condition", "error in"=w560, "Data In"=w550, "Func_ext"=w581) -> ("error out"=w556:errorcluster, "Func_ext Out"=w555:string)  [unwired: 5 in, 1 out]
        n289 = call "Variables Data IO.vi"("Select"=Cmd_Var_Data_IO."CMC Default", "error in"=w556, "Func_ext"=w555) -> ("error out"=w554:errorcluster, "Data Out"=w579:string[][], "Func_ext Out"=w553:string)  [unwired: 6 in]
        n290 = Build Array(w592, w593, w590, w589) -> (w591:refnum<vi>[])
        n291 = call "Variables Data IO.vi"("Select"=Cmd_Var_Data_IO."Spec Temp", "error in"=w554, "Func_ext"=w553) -> ("error out"=w552:errorcluster, "Data Out"=w562:string[][], "Func_ext Out"=w551:string)  [unwired: 6 in]
        n292 = call "Set State Controls.vi"("활성화 (F)"=TRUE, "컨트롤 참조 배열 in"=w591) -> ()  [unwired: 8 in, 2 out]
        n293 = call "STD Cal Data_etc.vi"("error in"=w552, "Func_ext"=w551) -> ("error out"=w559:errorcluster, "Data Out"=w549:string[][], "Func_ext Out"=w548:string)  [unwired: 5 in, 2 out]
        n294 = call "Get Spec.vi"("NumRows"=u32 28, "Spec in"=w562, "Spec Ref."=w595, "error in"=w559, "Condition in"=w550, "Resolution in"=w549, "Func_ext"=w548) -> ("error out"=w557:errorcluster, "Data Out"=w565:string[][], "Func_ext Out"=w558:string)  [unwired: 2 out]
        n295 = call "Match_CMC.vi"("CMC IN"=w579, "error in"=w557, "Condition IN"=w565, "Func_ext"=w558) -> ("error out"=w588:errorcluster, "Func_ext out"=w587:string)  [unwired: 4 in, 2 out]
        n296 = Index Array(array=w550, index (col)=0 ("비활성화된 인덱스 (열)")) -> (element=w566:string[])  [unwired: 1 in]
        n297 = call "Variables Data IO.vi"("Select"=w586, "error in"=w588, "Func_ext"=w587) -> ("error out"=w574:errorcluster, "Data Out"=w573:string[][], "Func_ext Out"=w572:string)  [unwired: 6 in]
        n298 = call "Variables Data IO.vi"("Select"=w569, "error in"=w574, "Func_ext"=w572) -> ("error out"=w571:errorcluster, "Data Out"=w568:string[][], "Func_ext Out"=w570:string)  [unwired: 6 in]
        n299 = for {
          tunnel: w550 -> [w612] mode=indexing
          tunnel: w573 -> [w609]
          shift-right: [w608] -> w584
          shift-left: string[][] [] -> [w606]
          tunnel: [w602] -> w576 mode=indexing
          tunnel: w568 -> [w601]
          tunnel: w566 -> [w600]
          i -> [w603]
          n300 = Index Array(array=w612) -> (element=w599:string)  [unwired: 1 in]
          n301 = Index Array(array=w609) -> (element=w611:string[])  [unwired: 2 in]
          n302 = Search 1D Array(1D array=w600, element=w599) -> (index of element=w598:i32)  [unwired: 1 in]
          n303 = Search 1D Array(1D array=w611, element=w599) -> (index of element=w610:i32)  [unwired: 1 in]
          n304 = case shown="-1" w610 {
            selector: w610 -> [w617 _]
            tunnel: w609 -> [w619 _]
            tunnel: [w618 w622] -> w607
            tunnel: w599 -> [_ w623]
            tunnel: [w613 string[] ["", "", "", ""]] -> w602
            tunnel: w601 -> [w615 _]
            tunnel: w598 -> [w614 _]
            frame Default {
              n305 = Index Array(array=w615, index (row)=w614) -> (element=w613:string[])  [unwired: 1 in]
              n306 = Delete From Array(array=w619, length=3 ("길이"), index (col)=w617) -> (deleted portion=w618:string[][])  [unwired: 1 in, 1 out]
            }
            frame -1 {
              w624 = 0 ("인덱스 (행)")
              n307 = Replace Array Subset(array=string[][] [["", "", ""], ["", "", ""], ["", "", ""], ["", "", ""], ["", "", ""], ["", "", ""], ["", "", ""], ["", "", ""], ["", "", ""], ["", "", ""], ["", "", ""], ["", "", ""], ["", "", ""]], new element=w623, index (row)=w624, index (col)=w624) -> (w622:string[][])
            }
          }
          n308 = Multiply(x=w603, y=3) -> (x*y=w604:i32)
          n309 = Insert Into Array(array=w606, index (col)=w604, new element=w607) -> (w608:string[][])  [unwired: 1 in]
        }
        n310 = call "Variables Data IO.vi"("Select"=w569, "error in"=w571, "Data In"=w576, "Func_ext"=w570) -> ("error out"=w577:errorcluster, "Func_ext Out"=w575:string)  [unwired: 5 in, 1 out]
        n311 = call "Variables Data IO.vi"("Select"=w586, "error in"=w577, "Data In"=w584, "Func_ext"=w575) -> ("error out"=w578:errorcluster)  [unwired: 5 in, 2 out]
      }
      frame "분동등급변경" {
        w632 = Cmd_Var_Data_IO."Result_Temp" ("Select")
        n312 = local read "시험분동"() -> (w626:i32)
        n313 = local read "분동등급"() -> (w628:string)
        n314 = call "Variables Data IO.vi"("Select"=w632, "error in"=w627, "Func_ext"=w635) -> ("error out"=w634:errorcluster, "Data Out"=w630:string[][], "Func_ext Out"=w633:string)  [unwired: 6 in]
        n315 = control-ref of="Measured"() -> (w642:refnum<vi>)
        n316 = control-ref of="편심오차"() -> (w643:refnum<vi>)
        n317 = control-ref of="Header2"() -> (w644:refnum<vi>)
        n318 = control-ref of="X=S-T"() -> (w645:refnum<vi>)
        n319 = case shown="참" "일괄\n변경" {
          tunnel: w630 -> [w651 w654]
          tunnel: [w650 w653] -> w629
          tunnel: w628 -> [w648 w652]
          tunnel: w626 -> [w647 _]
          frame False {
            n320 = Replace Array Subset(array=w651, new element=w648, index (row)=w647, index (col)=3 ("인덱스")) -> (w650:string[][])
          }
          frame True {
            n321 = for {
              tunnel: w654 -> [w658] mode=indexing
              tunnel: w652 -> [w657]
              tunnel: [w656] -> w653 mode=indexing
              n322 = Replace Array Subset(array=w658, new element=w657, index=3 ("인덱스")) -> (w656:string[])
            }
          }
        }
        n323 = call <vilib>:"Trim Whitespace.vi"("string"=w628) -> ("trimmed string"=w640:string)  [unwired: 1 in]
        n324 = Empty String/Path?(string/path=w640) -> (empty?=w639:bool)
        n325 = Build Array(w642, w643, w644, w645) -> (w641:refnum<vi>[])
        n326 = Select(t=FALSE, s=w639, f=TRUE) -> (s? t:f=w636:bool)
        n327 = call "Set State Controls.vi"("활성화 (F)"=w636, "컨트롤 참조 배열 in"=w641) -> ()  [unwired: 8 in, 2 out]
        n328 = call "Variables Data IO.vi"("Select"=w632, "error in"=w634, "Data In"=w629, "Func_ext"=w633) -> ("error out"=w631:errorcluster)  [unwired: 5 in, 2 out]
      }
    }
  }
  n329 = Release Queue(queue=w10, error in (no error)=w11) -> (error out=w8:errorcluster)  [unwired: 1 in, 2 out]
  n330 = Merge Errors(w9, w8) -> (→"에러 출력":errorcluster)
